vi "Check Parallel Gains.vi"(0 "proportional gain in":sgl, 5 "integral gain in (0)":sgl, 7 "derivative gain in (0)":sgl, 9 "filter coefficient in (0)":sgl, 11 "error in (no error)":errorcluster, 12 "sampling time":sgl) -> (4 "proportional gain out":sgl, 6 "integral gain out":sgl, 8 "derivative gain out":sgl, 10 "filter coefficient out":sgl, 15 "error out":errorcluster)   [LabVIEW 2017]
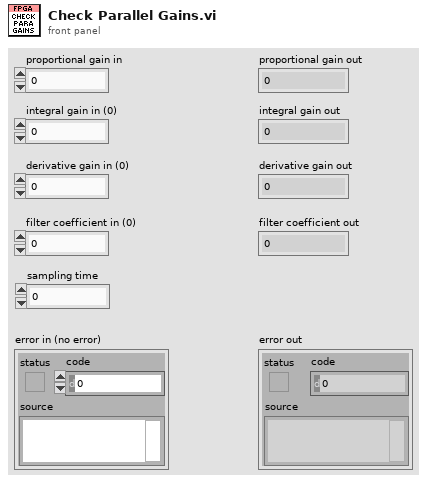
[diagram p1: front panel]
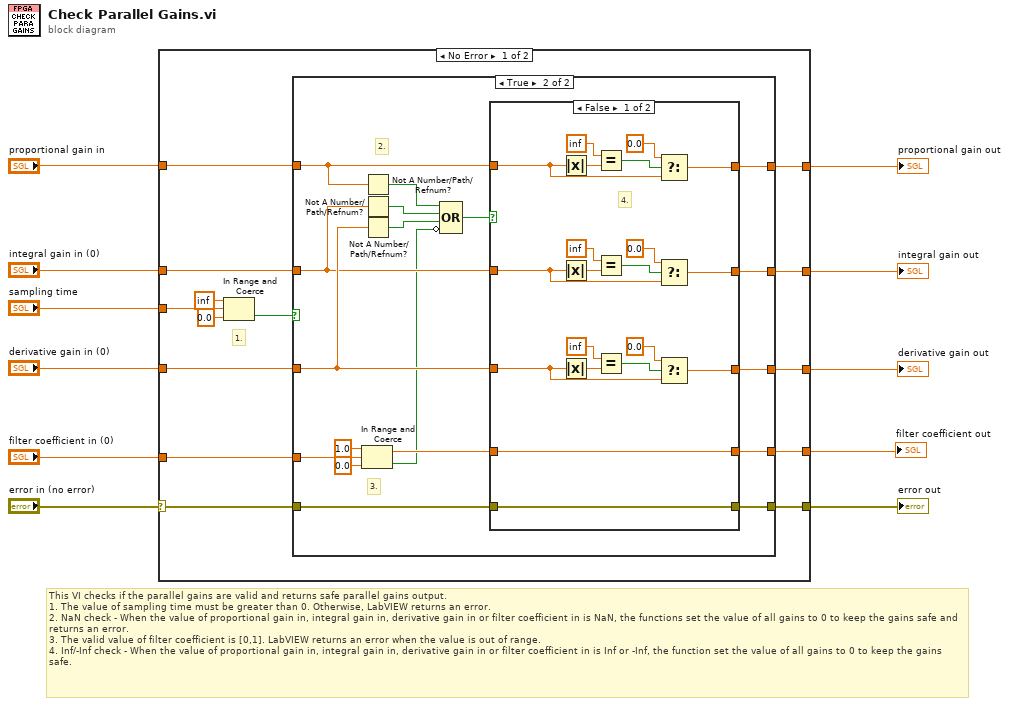
[diagram p0: block diagram]
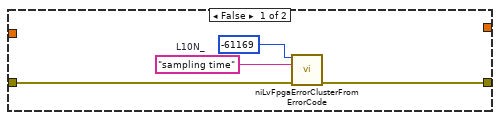
[diagram p2: hidden frame]
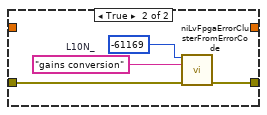
[diagram p3: hidden frame]
diagram:
  # "This VI checks if the parallel gains are valid and returns safe parallel gains output.\n1. The value of sampling time must be greater than 0. Otherwise, LabVIEW returns an error.\n2. NaN check - When the value of proportional gain in, integral gain in, derivative gain in or filter coefficient in is NaN, the functions set the value of all gains to 0 to keep the gains safe and returns an error.\n3. The valid value of filter coefficient is [0,1]. LabVIEW returns an error when the value is out of range.\n4. Inf/-Inf check - When the value of proportional gain in, integral gain in, derivative gain in or filter coefficient in is Inf or -Inf, the function set the value of all gains to 0 to keep the gains safe."
  n1 = case shown="No Error" "error in (no error)" {
    selector: "error in (no error)" -> [w25 w72]
    tunnel: "proportional gain in" -> [w18 _]
    tunnel: "integral gain in (0)" -> [w17 _]
    tunnel: "derivative gain in (0)" -> [w19 _]
    tunnel: "filter coefficient in (0)" -> [w16 _]
    tunnel: [w24 w72] -> w6
    tunnel: [w23 _] -> w5
    tunnel: [w22 _] -> w4
    tunnel: [w21 _] -> w3
    tunnel: [w20 _] -> w2
    tunnel: "sampling time" -> [w13 _]
    frame No Error {
      # "1."
      n2 = In Range and Coerce(upper limit=sgl inf, x=w13, lower limit=sgl 0.0) -> (In Range?=w12:bool)  [unwired: 1 out]
      n3 = case shown="True" w12 {
        tunnel: w25 -> [w27 w43]
        tunnel: [w26 w42] -> w24
        tunnel: [_ w41] -> w23
        tunnel: [_ w40] -> w22
        tunnel: [_ w39] -> w21
        tunnel: [_ w38] -> w20
        tunnel: w19 -> [_ w37]
        tunnel: w18 -> [_ w36]
        tunnel: w17 -> [_ w35]
        tunnel: w16 -> [_ w32]
        frame False {
          w28 = "sampling time"  # L10N_
          n4 = call <vilib>:"niLvFpgaErrorClusterFromErrorCode.vi"("error code"=-61169, "function name"=w28, "error in"=w27) -> ("error out"=w26:errorcluster)  [unwired: 4 in, 8 out]
        }
        frame True {
          # "3."
          # "2."
          n5 = In Range and Coerce(upper limit=sgl 1.0, x=w32, lower limit=sgl 0.0) -> (coerced(x)=w31:sgl, In Range?=w30:bool)
          n6 = Not A Number/Path/Refnum?(number/path/refnum=w36) -> (NaN/Path/Refnum?=w47:bool)
          n7 = Not A Number/Path/Refnum?(number/path/refnum=w35) -> (NaN/Path/Refnum?=w46:bool)
          n8 = Not A Number/Path/Refnum?(number/path/refnum=w37) -> (NaN/Path/Refnum?=w45:bool)
          n9 = Compound Arithmetic op=OR(w47, w46, w45, invert w30) -> (w44:bool)
          n10 = case shown="False" w44 {
            tunnel: w36 -> [w67 _]
            tunnel: w35 -> [w66 _]
            tunnel: w37 -> [w61 _]
            tunnel: w31 -> [w48 _]
            tunnel: [w65 _] -> w38
            tunnel: [w64 _] -> w39
            tunnel: [w63 _] -> w40
            tunnel: [w48 _] -> w41
            tunnel: w43 -> [w62 w70]
            tunnel: [w62 w69] -> w42
            frame False {
              # "4."
              n11 = Absolute Value(x=w67) -> (abs(x)=w50:sgl)
              n12 = Absolute Value(x=w66) -> (abs(x)=w54:sgl)
              n13 = Absolute Value(x=w61) -> (abs(x)=w58:sgl)
              n14 = Equal?(x=sgl inf ("y"), y=w50) -> (x = y?=w51:bool)
              n15 = Equal?(x=sgl inf ("y"), y=w54) -> (x = y?=w55:bool)
              n16 = Equal?(x=sgl inf ("y"), y=w58) -> (x = y?=w59:bool)
              n17 = Select(t=sgl 0.0, s=w51, f=w67) -> (s? t:f=w65:sgl)
              n18 = Select(t=sgl 0.0, s=w55, f=w66) -> (s? t:f=w64:sgl)
              n19 = Select(t=sgl 0.0, s=w59, f=w61) -> (s? t:f=w63:sgl)
            }
            frame True {
              w68 = "gains conversion"  # L10N_
              n20 = call <vilib>:"niLvFpgaErrorClusterFromErrorCode.vi"("error code"=-61169, "function name"=w68, "error in"=w70) -> ("error out"=w69:errorcluster)  [unwired: 4 in, 8 out]
            }
          }
        }
      }
    }
    frame Error {
    }
  }
  "proportional gain out" <- w2
  "integral gain out" <- w3
  "derivative gain out" <- w4
  "filter coefficient out" <- w5
  "error out" <- w6
